vi "TDMS Reference Create.vi"(8 "error in (no error)":errorcluster, 9 "FileName":string, 11 "Refs":T1) -> (0 "error out":errorcluster, 3 "Refs Out":T1)   [LabVIEW 2020]
uses:
  controls/UI Data.ctl
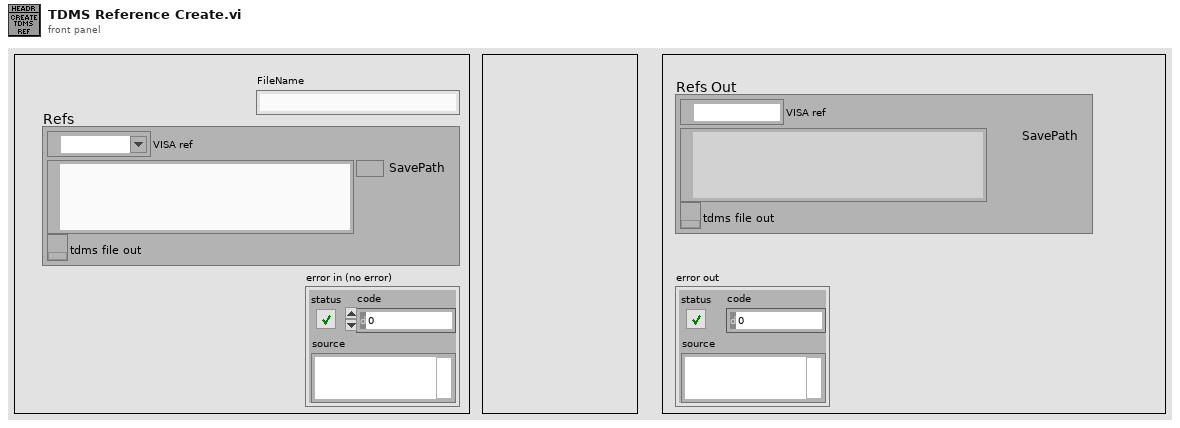
[diagram p1: front panel]
types:
  T1 = typedef "UI Data.ctl" = cluster{"VISA ref":refnum<visa-resource-name>, "SavePath":path, "tdms file out":refnum<k34>}
  T2 = enum16{"open", "open or create", "create or replace", "create", "open (read-only)"}
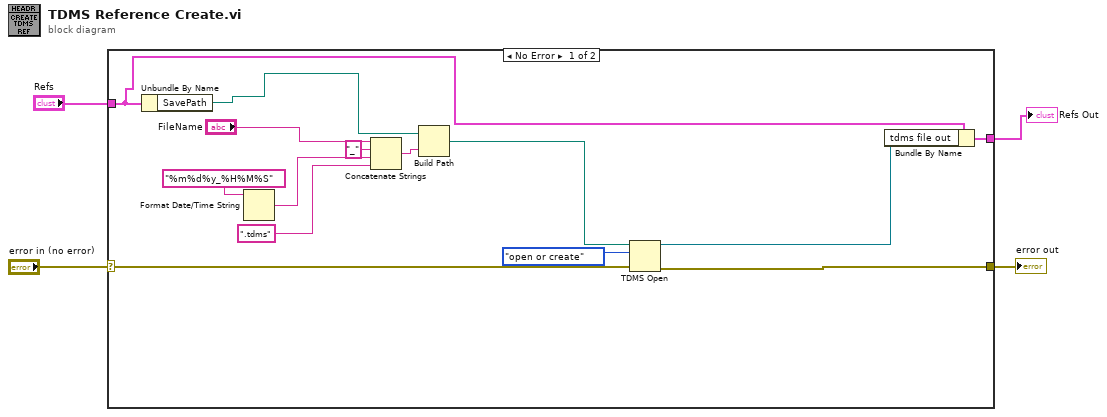
[diagram p0: block diagram]
diagram:
  n1 = case shown="No Error" "error in (no error)" {
    selector: "error in (no error)" -> [w13 w20]
    tunnel: [w16 w20] -> w4
    tunnel: "Refs" -> [w11 w19]
    tunnel: [w9 w19] -> w1
    frame No Error {
      n2 = Unbundle By Name(w11) -> ("SavePath"=w12:path)
      n3 = Format Date/Time String(time format string (%c)="%m%d%y_%H%M%S") -> (date/time string=w8:string)  [unwired: 2 in]
      n4 = Concatenate Strings("FileName", "_" ("string"), w8, ".tdms" ("string")) -> (w17:string)
      n5 = Build Path(base path=w12, name or relative path=w17) -> (appended path=w18:path)
      n6 = TDMS Open(8:w13, 10:T2."open or create" ("operation (0:open)"), 11:w18) -> (0:w16:errorcluster, 3:w10:refnum<k34>)  [unwired: 4 in]
      n7 = Bundle By Name(cluster=w11, "tdms file out"=w10) -> (w9:T1)
    }
    frame Error {
    }
  }
  "error out" <- w4
  "Refs Out" <- w1
